vi "error generator.vi"(5 "error (T)":bool=TRUE, 6 "error in":errorcluster, 7 "source":string="error generator.vi", 8 "append error message":string, 9 "error code (0)":i32) -> (0 "error out":errorcluster)   [LabVIEW 2013, in "NISE_CEF_TreeControl.lvlib"]
doc: "Converts an error or warning code to an error cluster. This VI is useful when you receive a return value from a shared library call or when you return user-defined error codes."
uses:
  NISE_CEF_TreeControl.lvlib
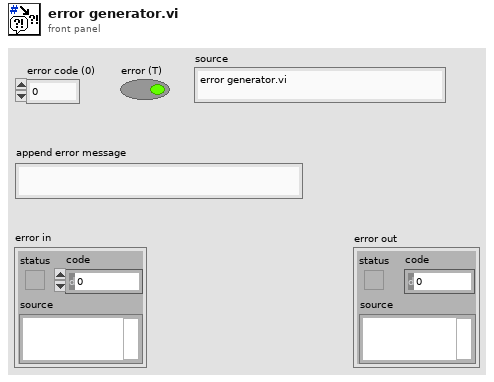
[diagram p1: front panel]
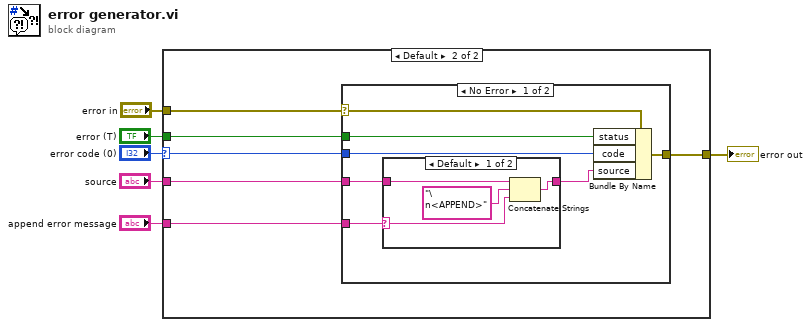
[diagram p0: block diagram]
diagram:
  n1 = case shown="Default" "error code (0)" {
    selector: "error code (0)" -> [_ w11]
    tunnel: "error in" -> [w7 w13]
    tunnel: [w7 w12] -> w4
    tunnel: "source" -> [_ w10]
    tunnel: "append error message" -> [_ w9]
    tunnel: "error (T)" -> [_ w8]
    frame 0 {
      # "If the error code in equals zero, then propagate the error in cluster regardless of its value."
    }
    frame Default {
      n2 = case shown="No Error" w13 {
        selector: w13 -> [w18 w26]
        tunnel: [w19 w26] -> w12
        tunnel: w11 -> [w20 _]
        tunnel: w10 -> [w15 _]
        tunnel: w9 -> [w17 _]
        tunnel: w8 -> [w14 _]
        frame No Error {
          n3 = case shown="Default" w17 {
            selector: w17 -> [w22 _]
            tunnel: [w21 w25] -> w16
            tunnel: w15 -> [w24 w25]
            frame Default {
              n4 = Concatenate Strings(w24, "\n<APPEND>" ("string"), w22) -> (w21:string)
            }
            frame "" {
            }
          }
          n5 = Bundle By Name(cluster=w18, "status"=w14, "code"=w20, "source"=w16) -> (w19:errorcluster)
        }
        frame Error {
          # "An error in trumps any error code input."
        }
      }
    }
  }
  "error out" <- w4
